vi "TDMSAdv writeOfVar.vi"(5 "channel name":string, 7 "group name (Untitled)":string, 8 "error in (no error)":errorcluster, 10 "dataArray":variant[](array[variant]), 11 "TDMSAdv in":refnum<class "TDMSAdv.lvclass">) -> (0 "error out":errorcluster, 3 "TDMSAdv out":refnum<class "TDMSAdv.lvclass">)   [LabVIEW 2018, in "TDMSAdv.lvclass"]
uses:
  TDMSAdv.lvclass
  <vilib>/Utility/error.llb/Error Cluster From Error Code.vi
  <vilib>/ErrorRing/Error Ring.xnode
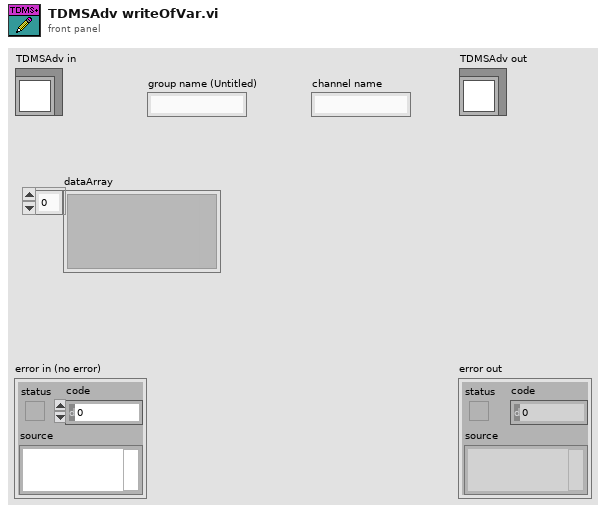
[diagram p1: front panel]
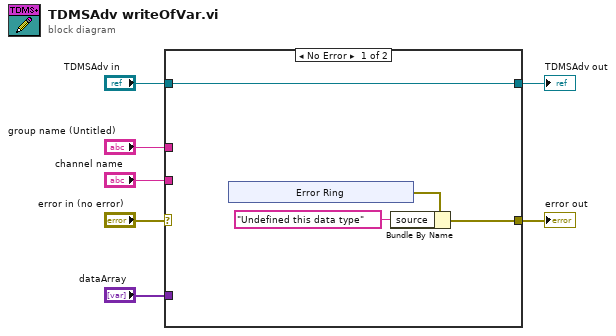
[diagram p0: block diagram]
diagram:
  n1 = case shown="No Error" "error in (no error)" {
    selector: "error in (no error)" -> [_ w16]
    tunnel: "group name (Untitled)" -> [_ _]
    tunnel: "channel name" -> [_ _]
    tunnel: "TDMSAdv in" -> [w11 w17]
    tunnel: [w11 w17] -> w4
    tunnel: [w8 w16] -> w3
    tunnel: "dataArray" -> [_ _]
    frame No Error {
      n2 = xnode "Error Ring"() -> ("error out"=w10:errorcluster)
      n3 = Bundle By Name(cluster=w10, "source"="Undefined this data type") -> (w8:errorcluster)
    }
    frame Error {
    }
  }
  "TDMSAdv out" <- w4
  "error out" <- w3
